vi "Write X column ref.vi"(8 "error in (no error)":errorcluster, 10 "X column ref":refnum<vi>, 11 "XY WFRM Plot in":refnum<class "XY WFRM Plot.lvclass">) -> (0 "error out":errorcluster, 3 "XY WFRM Plot out":refnum<class "XY WFRM Plot.lvclass">)   [LabVIEW 2018, in "XY WFRM Plot.lvclass"]
uses:
  XY WFRM Plot.lvclass
  XY WFRM Plot.lvclass/XY WFRM Plot.ctl
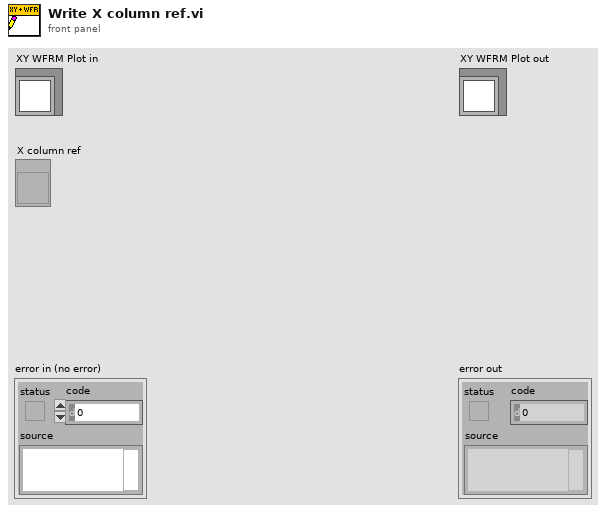
[diagram p1: front panel]
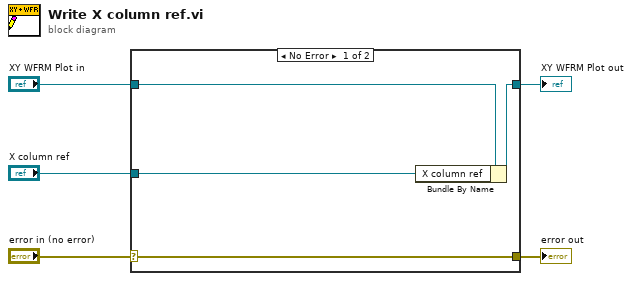
[diagram p0: block diagram]
diagram:
  n1 = case shown="No Error" "error in (no error)" {
    selector: "error in (no error)" -> [w9 w10]
    tunnel: [w9 w10] -> w4
    tunnel: [w7 w11] -> w2
    tunnel: "XY WFRM Plot in" -> [w8 w11]
    tunnel: "X column ref" -> [w6 _]
    frame No Error {
      n2 = Bundle By Name(cluster=w8, "X column ref"=w6) -> (w7:refnum<class "XY WFRM Plot.lvclass">)
    }
    frame Error {
    }
  }
  "error out" <- w4
  "XY WFRM Plot out" <- w2
